vi "Get First Pad Byte.vi"(1 "Hash Function":refnum<class "NI_SHA-3.lvclass">) -> (0 "first pad byte":u8=6)   [LabVIEW 2020, in "NI_SHA-3.lvclass"]
doc: "Returns the message padding associated with this Keccak variant, along with the leading bit of pad10*1."
uses:
  <vilib>/security/Message Digest/SHA-3/NI_SHA-3.lvclass
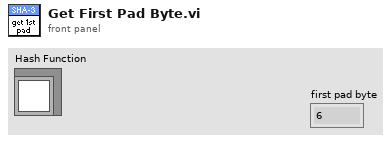
[diagram p1: front panel]
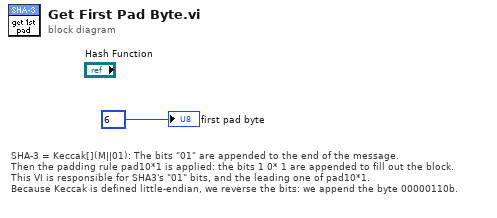
[diagram p0: block diagram]
diagram:
  # "SHA-3 = Keccak[](M||01): The bits \"01\" are appended to the end of the message.\nThen the padding rule pad10*1 is applied: the bits 1 0* 1 are appended to fill out the block.\nThis VI is responsible for SHA3's \"01\" bits, and the leading one of pad10*1.\nBecause Keccak is defined little-endian, we reverse the bits: we append the byte 00000110b."
  "first pad byte" <- u8 6 ("first pad byte mask")
